vi "MakeCircles.vi"(10 "Y":dbl[](array[numeric])=[4.0, 2.0, 7.0, 6.0], 11 "X":dbl[](array[numeric])=[2.0, 5.0, 7.0, 3.0]) -> (3 "Circles cluster":cluster{dbl[], dbl[]})   [LabVIEW 2019]
panel:
  in  "Radius":dbl=100.0
  out "XY Graph":cluster{"X":dbl[], "Y":dbl[]}[](graph)
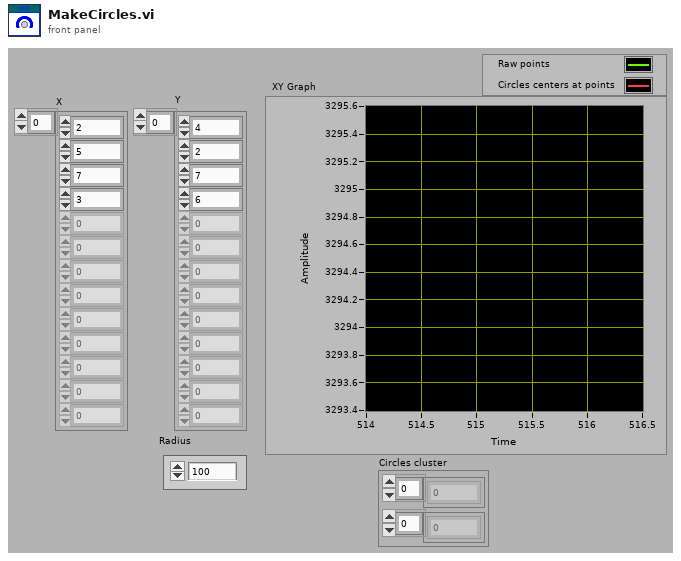
[diagram p1: front panel]
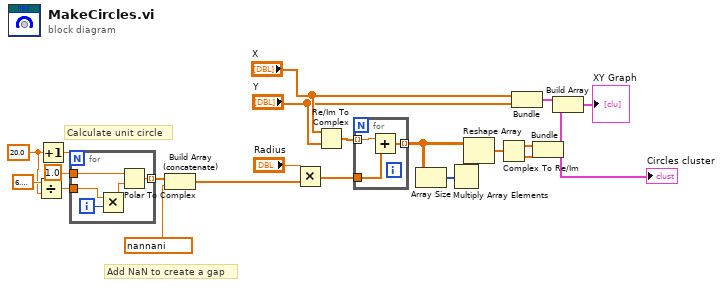
[diagram p0: block diagram]
diagram:
  w19 = 20.0
  # "Calculate unit circle"
  # "Add NaN to create a gap"
  n1 = Divide(x=6.283185307179586, y=w19) -> (x/y=w18:dbl)
  n2 = Increment(x=w19) -> (x+1=w21:dbl)
  n3 = for {
    N: w21 -> [_]
    tunnel: 1.0 ("r") -> [w27]
    tunnel: w18 -> [w25]
    tunnel: [w23] -> w17 mode=indexing
    i -> [w26]
    n4 = Multiply(x=w25, y=w26) -> (x*y=w24:dbl)
    n5 = Polar To Complex(1:w24, 2:w27) -> (0:w23:cdb)
  }
  n6 = Build Array (concatenate)(w17, cdb nan+nani) -> (w15:cdb[])
  n7 = Multiply(x="Radius", y=w15) -> (x*y=w12:cdb[])
  n8 = Re/Im To Complex(1:"Y", 2:"X") -> (0:w9:cdb[])
  n9 = for {
    tunnel: w12 -> [w29]
    tunnel: w9 -> [w30] mode=indexing
    tunnel: [w28] -> w7 mode=indexing
    n10 = Add(x=w30, y=w29) -> (x+y=w28:cdb[])
  }
  n11 = Array Size(array=w7) -> (size(s)=w6:i32[])
  n12 = Multiply Array Elements(1:w6) -> (0:w5:i32)
  n13 = Reshape Array(w7, w5) -> (w4:cdb[])
  n14 = Complex To Re/Im(x + iy=w4) -> (x=w3:dbl[], y=w2:dbl[])
  n15 = Bundle("X"="X", "Y"="Y") -> (w14:cluster{"X":dbl[], "Y":dbl[]})  [unwired: 1 in]
  n16 = Bundle(w3, w2) -> (w1:cluster{dbl[], dbl[]})  [unwired: 1 in]
  "Circles cluster" <- w1
  n17 = Build Array(w14, w1) -> (→"XY Graph":cluster{"X":dbl[], "Y":dbl[]}[])
